vi "Get Image.vi"(7 "Offset":T2, 8 "Error In":errorcluster, 9 "Mouse-over":bool, 10 "Selected":bool, 11 "Panel Object in":refnum<class "Panel Object.lvclass">) -> (0 "Error Out":errorcluster, 2 "Image":T1, 3 "Panel Object out":refnum<class "Panel Object.lvclass">)   [LabVIEW 2015, in "Panel Object.lvclass"]
uses:
  Panel Object.lvclass
  Typedefs/Point--Cluster.ctl
  <vilib>/picture/picture.llb/imagedata.ctl
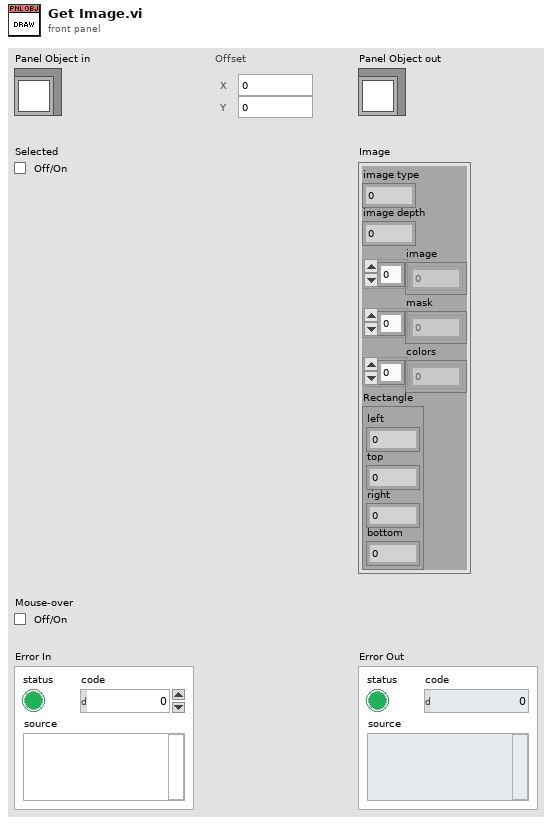
[diagram p1: front panel]
types:
  T1 = typedef "imagedata.ctl" = cluster{"image type":i32, "image depth":i32, "image":u8[], "mask":u8[], "colors":u32[], "Rectangle":cluster{"left":i16, "top":i16, "right":i16, "bottom":i16}}
  T2 = typedef "Point--Cluster.ctl" = cluster{"Horizontal":i32, "Vertical":i32}
  T3 = cluster{"left":i16, "top":i16, "right":i16, "bottom":i16}
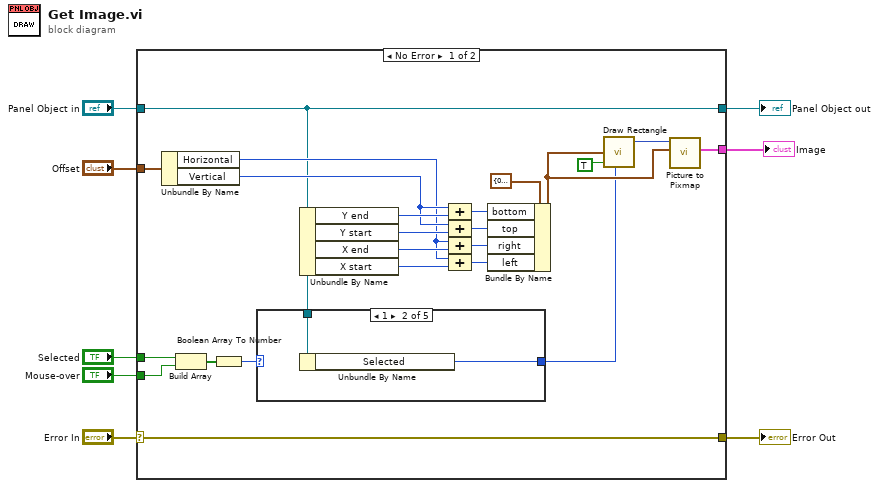
[diagram p0: block diagram]
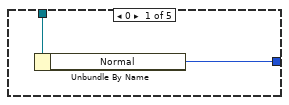
[diagram p2: hidden frame]
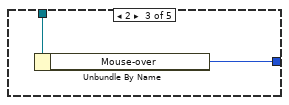
[diagram p3: hidden frame]
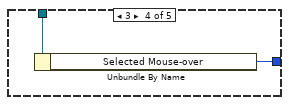
[diagram p4: hidden frame]
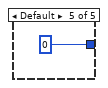
[diagram p5: hidden frame]
diagram:
  n1 = case shown="No Error" "Error In" {
    selector: "Error In" -> [w31 w42]
    tunnel: [w31 w42] -> w5
    tunnel: [w12 w41] -> w7
    tunnel: "Panel Object in" -> [w12 w41]
    tunnel: "Offset" -> [w22 _]
    tunnel: [w17 _] -> w3
    tunnel: "Selected" -> [w9 _]
    tunnel: "Mouse-over" -> [w10 _]
    frame No Error {
      n2 = Unbundle By Name(w22) -> ("Horizontal"=w19:i32, "Vertical"=w21:i32)
      n3 = Build Array(w9, w10) -> (w14:bool[])
      n4 = Boolean Array To Number(Boolean array=w14) -> (number=w13:u32)
      n5 = case shown="1" w13 {
        tunnel: w12 -> [w33 w35 w37 w39 _]
        tunnel: [w32 w34 w36 w38 u32 0 ("Selected Mouse-over")] -> w11
        frame 0 {
          n6 = Unbundle By Name(w33) -> ("Normal"=w32:u32)
        }
        frame 1 {
          n7 = Unbundle By Name(w35) -> ("Selected"=w34:u32)
        }
        frame 2 {
          n8 = Unbundle By Name(w37) -> ("Mouse-over"=w36:u32)
        }
        frame 3 {
          n9 = Unbundle By Name(w39) -> ("Selected Mouse-over"=w38:u32)
        }
        frame Default {
        }
      }
      n10 = Unbundle By Name(w12) -> ("Y end"=w29:i32, "Y start"=w28:i32, "X end"=w27:i32, "X start"=w20:i32)
      n11 = Compound Arithmetic op=ADD(w21, w29) -> (w26:i32)
      n12 = Compound Arithmetic op=ADD(w21, w28) -> (w25:i32)
      n13 = Compound Arithmetic op=ADD(w19, w27) -> (w24:i32)
      n14 = Compound Arithmetic op=ADD(w19, w20) -> (w23:i32)
      n15 = Bundle By Name(cluster=T3 {"left"=0, "top"=0, "right"=0, "bottom"=0} ("rect"), "bottom"=w26, "top"=w25, "right"=w24, "left"=w23) -> (w15:T3)
      n16 = call <vilib>:"Draw Rectangle.vi"("rect"=w15, "fill?(F)"=TRUE, "color(black)"=w11) -> ("new picture"=w18:picture)  [unwired: 6 in]
      n17 = call <vilib>:"Picture to Pixmap.vi"("rect"=w15, "picture"=w18) -> ("image data"=w17:T1)  [unwired: 8 in, 1 out]
    }
    frame Error {
    }
  }
  "Panel Object out" <- w7
  "Error Out" <- w5
  "Image" <- w3
